vi "DC - Data setup acquisition.vi"(1 "Setup data acquisition in the following syntax:\nnn1 - data acquisition mode,\nnn2 - axis used to trigger data acquisition,\nnn3 - data acquisition parameter 3,\nnn4 - data acquisition parameter 4,\nnn5 - data acquisition rate,\nnn6 - number of data samples to be acquired":string, 2 "error in":errorcluster, 3 "Address / Port":i16=1 min=1 max=31 step=1) -> (0 "error out":errorcluster)   [LabVIEW 2014]
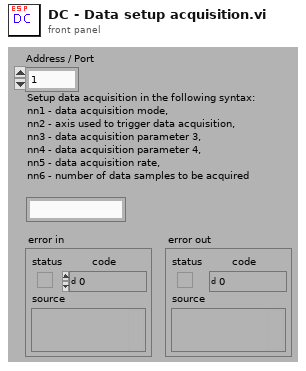
[diagram p1: front panel]
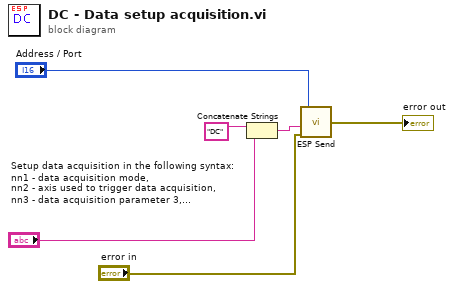
[diagram p0: block diagram]
diagram:
  n1 = Concatenate Strings("DC" ("Substring"), "Setup data acquisition in the following syntax:\nnn1 - data acquisition mode,\nnn2 - axis used to trigger data acquisition,\nnn3 - data acquisition parameter 3,\nnn4 - data acquisition parameter 4,\nnn5 - data acquisition rate,\nnn6 - number of data samples to be acquired") -> (w5:string)
  n2 = call "ESP Send.vi"("Address / Port"="Address / Port", "Command String"=w5, "error in"="error in") -> ("error out"=→"error out":errorcluster)  [unwired: 5 in]
